vi "Set DA Single.vi"(8 "error in (no error)":errorcluster caption="错误输入（无错误）", 9 "da_value":sgl, 10 "ch":i32, 11 "dev":i32) -> (0 "error out":errorcluster caption="错误输出", 3 "function return":i32)   [LabVIEW 2018, in "恒凯采集卡.lvlib"]
doc: "int Set_DA_Single(int dev,int ch,float da_value);"
uses:
  data/Usb_Daq_V52_32.dll
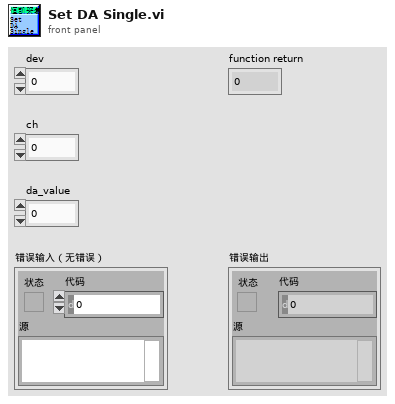
[diagram p1: front panel]
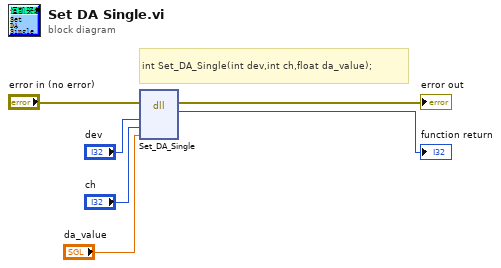
[diagram p0: block diagram]
diagram:
  # "int Set_DA_Single(int dev,int ch,float da_value);"
  n1 = dll-call lib="D:/ProgramFiles/NI/LabVIEW 2018/user.lib/Usb_Daq_V52_32/Usb_Daq_V52_32.*" fn="Set_DA_Single"(error in="error in (no error)", "dev"="dev", "ch"="ch", "da_value"="da_value") -> (error out=→"error out":errorcluster, →"function return":i32)  [unwired: 5 in, 1 out]
